vi "test single REQ v3.vi"() -> ()   [LabVIEW 2018, in "LV-0mq-Julia_roundtrip-lib.lvlib"]
uses:
  LV-0mq-Julia_roundtrip-lib.lvlib
  Commands.ctl
  commands LV2Jl.ctl
  example server response cluster.ctl
  dd99417b-9b2e-46cd-a2e6-0761ab186cd0.vi
  <vilib>/addons/zeromq/zmq_socket.lvclass
  Julia functions enum.ctl
panel:
  out "JSON data REQ 2":string="{\"fun2call\":\"myfunc\", \"arg1\":0, \"arg2\":3.1415}"
  in  "error in (no error)":errorcluster
  out "parsed response":T1={"bin_lng"=1, "a1"=1, "a2"=3.14}
  in  "fun2call":T2
  in  "Arguments":cluster{"arg1":i32, "arg2":dbl}={"arg1"=1, "arg2"=3.14}
  in  "use binary data":bool
  in  "binary data in":u8[](array[numeric])=[1, 2, 3, 4]
  out "JSON data REQ":string="{\"fun2call\":\"myfunc\", \"arg1\":0, \"arg2\":3.1415}"
  in  "Command":T3=99 items=["call function"=99, "ping"=112, "stop"=115, "unused"=254]
  out "short err code":u8
  out "roundtrip time":dbl
  out "detailed err description or other information":string
  out "JSON data":string
  out "binary data out":u8[](array[numeric])
  out "server response":string
  out "error out":errorcluster
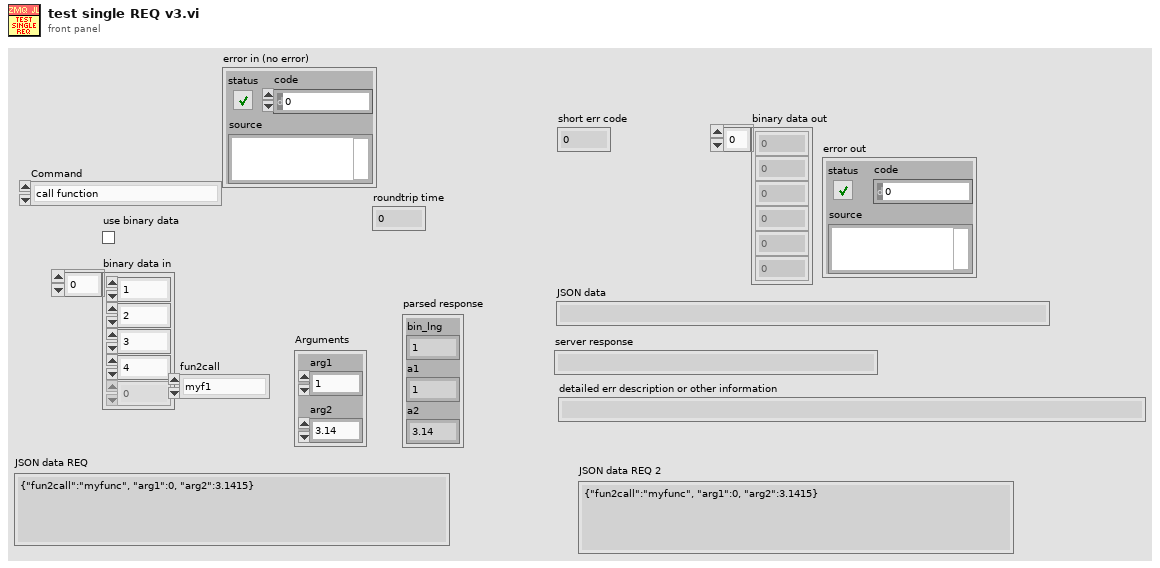
[diagram p1: front panel]
types:
  T1 = typedef "LV-0mq-Julia_roundtrip-lib.lvlib/example server response cluster.ctl" = cluster{"bin_lng":i32, "a1":i32, "a2":dbl}
  T2 = typedef "Julia functions enum.ctl" = enum16{"myf1", "myf2", "myf3", "test_bin2nums", "test_rgbimg", "numarr_loopback", "numarrs_lpbk", "Not_a_Fun"}
  T3 = typedef "LV-0mq-Julia_roundtrip-lib.lvlib/commands LV2Jl.ctl" = u8
  T4 = typedef "LV-0mq-Julia_roundtrip-lib.lvlib/Commands.ctl" = enum16{"Start Jl-server & Init LV-client", "Send request & Get response ", "Stop Jl-server & Cleanup LV-client", "Cleanup LV-client", "Start Jl-server", "Stop Jl-server", "Init LV-Client", "Cleanup LV-Client", "(not allowed)", "Set LV Client state", "Set Jl Server state", "set ZMQ timeout", "read ZMQ timeout", "read-out state"}
  T5 = typedef "LV-0mq-Julia_roundtrip-lib.lvlib/detailed error info.ctl" = cluster{"exception_or_info":string, "trace":T6[]}
  T6 = typedef "LV-0mq-Julia_roundtrip-lib.lvlib/StackFrame.ctl" = cluster{"frame_summary":string, "func":string, "linfo":string, "file":string, "line":i32, "pointer":u64, "from_c":bool, "inlined":bool}
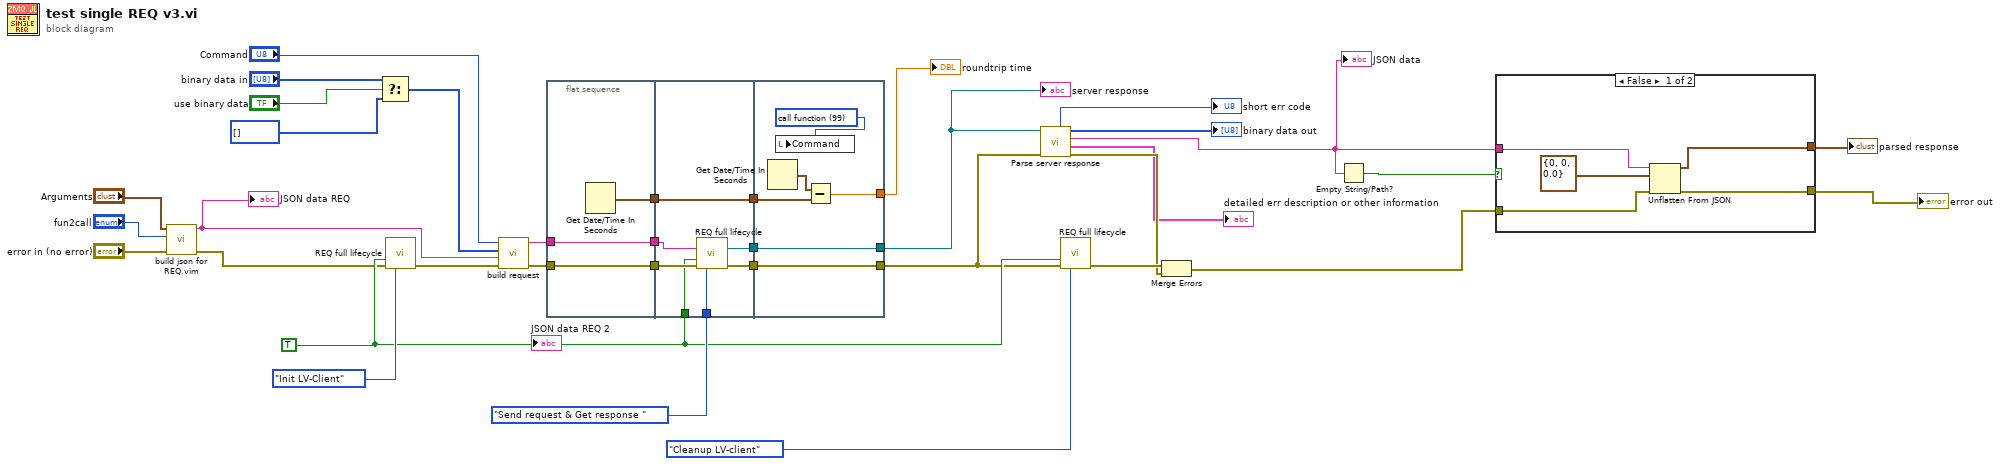
[diagram p0: block diagram]
diagram:
  w32 = TRUE ("Force command")
  n1 = call "build json for REQ.vim"("error in (no error)"="error in (no error)", "Arguments 2"="fun2call", "Arguments 1"="Arguments") -> ("error out"=w10:errorcluster, "JSON string out"=w1:string)  [unwired: 6 in, 1 out]
  "JSON data REQ" <- w1
  n2 = Select(t="binary data in", s="use binary data", f=u8[] [] ("binary data in 2")) -> (s? t:f=w12:u8[])
  n3 = call "REQ full lifecycle.vi"("Force command"=w32, "error in"=w10, "command"=Commands."Init LV-Client") -> ("error out"=w19:errorcluster)  [unwired: 6 in, 6 out]
  n4 = call "build request.vi"("error in (no error)"=w19, "JSON data"=w1, "binary data"=w12, "Command"="Command") -> ("error out"=w18:errorcluster, "REQ string"=w16:string)  [unwired: 6 in]
  n5 = flat-sequence {
    tunnel: w18 -> [w39]
    tunnel: [w39] -> w24
    tunnel: [w38] -> w23
    tunnel: [w37] -> w17
    tunnel: w16 -> [w37]
    tunnel: Commands."Send request & Get response " ("command") -> [w45]
    tunnel: w32 -> [w44]
    tunnel: [w43] -> w26
    tunnel: [w42] -> w25
    tunnel: w24 -> [w46]
    tunnel: w23 -> [w41]
    tunnel: [w41] -> w22
    tunnel: w17 -> [w40]
    tunnel: [w51] -> w30
    tunnel: [w52] -> w31
    tunnel: w26 -> [w52]
    tunnel: w25 -> [w51]
    tunnel: w22 -> [w49]
    tunnel: [w48] -> w21
    frame #0 {
      n6 = Get Date/Time In Seconds() -> (seconds since 1Jan1904=w38:timestamp)
    }
    frame #1 {
      n7 = call "REQ full lifecycle.vi"("data to send"=w40, "Force command"=w44, "error in"=w46, "command"=w45) -> ("socket out"=w43:refnum<class "zmq_socket.lvclass">, "error out"=w42:errorcluster)  [unwired: 5 in, 5 out]
    }
    frame #2 {
      w47 = T3 99 items=["call function"=99, "stop"=112] ("Command")
      n8 = Get Date/Time In Seconds() -> (seconds since 1Jan1904=w50:timestamp)
      n9 = local write "Command"(w47) -> ()
      n10 = Subtract(x=w50, y=w49) -> (x-y=w48:dbl)
    }
  }
  n11 = call "Parse server response.vi"("error in (no error)"=w30, "server response in"=w31) -> ("error out"=w29:errorcluster, "detailed error info"=→"detailed err description or other information":T5, "JSON out"=w7:string, "binary data"=→"binary data out":u8[], "return code"=→"short err code":u8)  [unwired: 2 in, 3 out]
  "JSON data" <- w7
  n12 = call "REQ full lifecycle.vi"("Force command"=w32, "error in"=w30, "command"=Commands."Cleanup LV-client") -> ("error out"=w34:errorcluster)  [unwired: 6 in, 6 out]
  n13 = Merge Errors(w34, w29) -> (w9:errorcluster)
  n14 = Empty String/Path?(string/path=w7) -> (empty?=w6:bool)
  n15 = case shown="False" w6 {
    tunnel: w7 -> [w57 _]
    tunnel: w9 -> [w56 w58]
    tunnel: [w55 w58] -> w8
    tunnel: [w54 _] -> w3
    frame False {
      n16 = Unflatten From JSON(JSON string=w57, type and defaults=T1 {"bin_lng"=0, "a1"=0, "a2"=0.0} ("parsed response"), error in (no error)=w56) -> (value=w54:T1, error out=w55:errorcluster)  [unwired: 4 in]
    }
    frame True {
    }
  }
  "error out" <- w8
  "parsed response" <- w3
  "server response" <- w31
  "roundtrip time" <- w21
